vi "Control_Twin_Source.vi"(0 "Control":T2(ring), 1 "Mode":T1) -> ()   [LabVIEW 2010]
uses:
  Controls/User_Specific_mode.ctl
  ADAM Client/Sub VIs/ADAM Controls/Update_scan_value.ctl
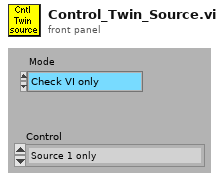
[diagram p1: front panel]
types:
  T1 = typedef "User_Specific_mode.ctl" = enum16{"Check VI only", "Run VI"}
  T2 = enum16{"Source 1 only", "Source 2 only", "Both Sources"}
  T3 = typedef "Update_scan_value.ctl" = cluster{"Channel Name":string, "New Value":dbl}
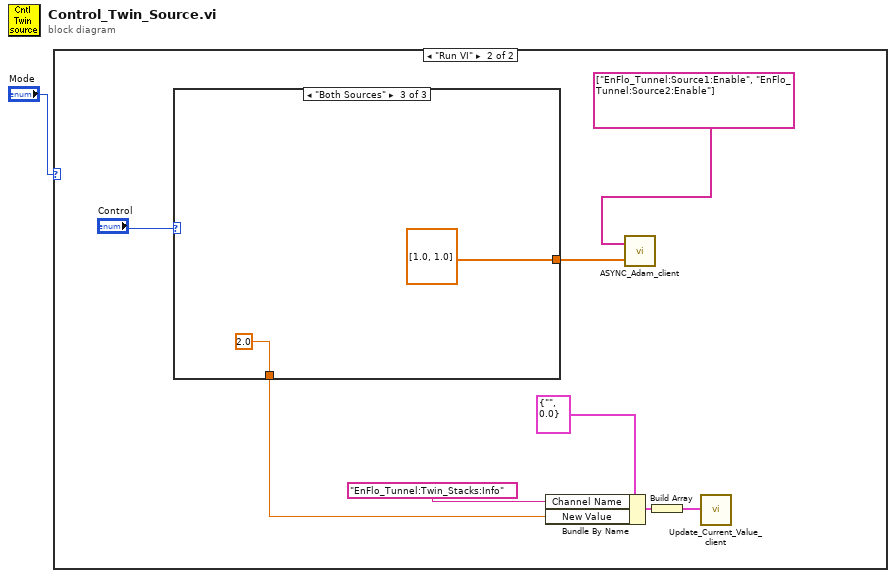
[diagram p0: block diagram]
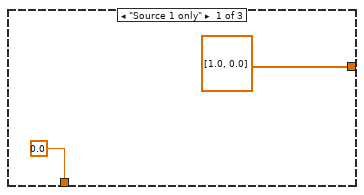
[diagram p3: hidden frame]
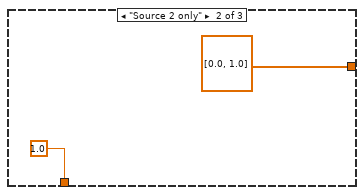
[diagram p4: hidden frame]
diagram:
  n1 = case shown="\"Run VI\"" "Mode" {
    frame "Check VI only" {
    }
    frame "Run VI" {
      n2 = case shown="\"Both Sources\"" "Control" {
        tunnel: [0.0 1.0 2.0] -> w4
        tunnel: [dbl[] [1.0, 0.0] ("Values") dbl[] [0.0, 1.0] ("Values") dbl[] [1.0, 1.0] ("Values")] -> w2
        frame "Source 1 only" {
        }
        frame "Source 2 only" {
        }
        frame "Both Sources" {
        }
      }
      n3 = Bundle By Name(cluster=T3 {"Channel Name"="", "New Value"=0.0} ("Update Scan Value Cluster"), "Channel Name"="EnFlo_Tunnel:Twin_Stacks:Info", "New Value"=w4) -> (w7:T3)
      n4 = call "ASYNC_Adam_client.vi"("Values"=w2, "Channel Names"=string[] ["EnFlo_Tunnel:Source1:Enable", "EnFlo_Tunnel:Source2:Enable"]) -> ()  [unwired: 2 out]
      n5 = Build Array(w7) -> (w6:T3[])
      n6 = call "Update_Current_Value_client.vi"("Update array in"=w6) -> ()  [unwired: 1 in]
    }
  }
